vi "DB - Array to Values.vi"(11 "Array (0xFFFE autodetect)":string[](array[string])) -> (3 "<Values>":string)   [LabVIEW 2020]
panel:
  # "abc\ndef\nghi\n(BOM)de"
  # "="
  # "'abc' ,'def' ,'ghi',CONVERT(varbinary(max),'0xFFFE6465',1)"
  # "BOM attached"
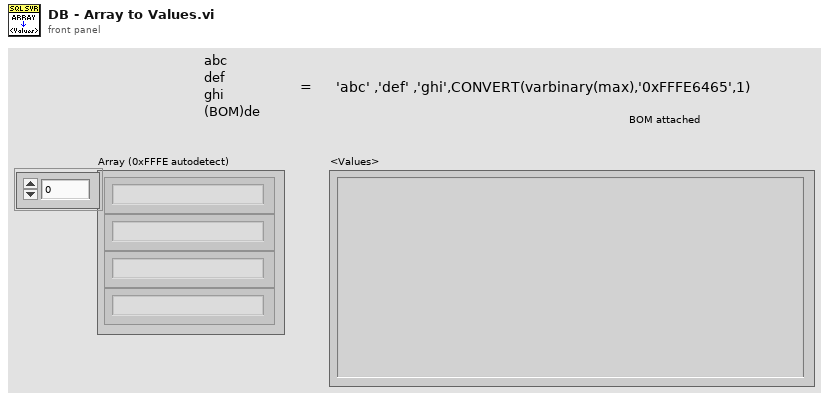
[diagram p1: front panel]
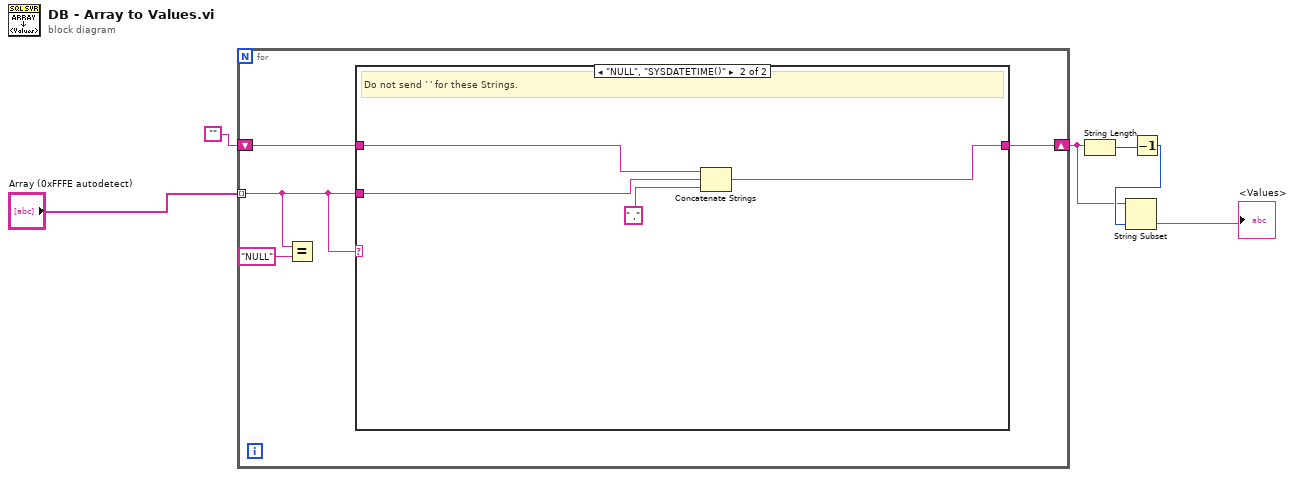
[diagram p0: block diagram]
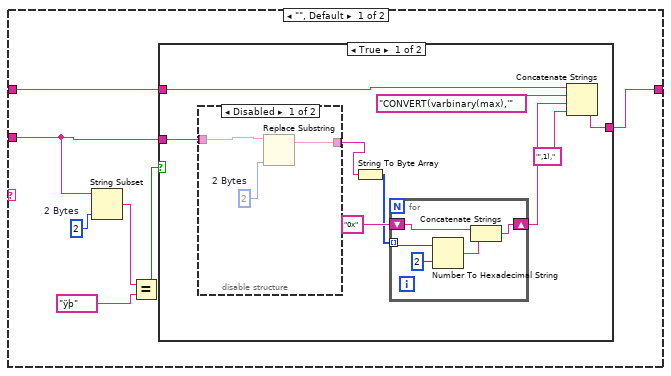
[diagram p2: hidden frame]
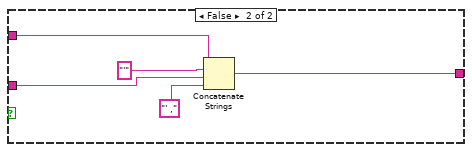
[diagram p4: hidden frame]
diagram:
  n1 = for {
    shift-right: [w9] -> w2
    shift-left: "" -> [w10]
    tunnel: "Array (0xFFFE autodetect)" -> [w7] mode=indexing
    n2 = Equal?(x=w7, y="NULL") -> ()  [unwired: 1 out]
    n3 = case shown="\"NULL\", \"SYSDATETIME()\"" w7 {
      tunnel: w10 -> [w17 w44]
      tunnel: [w16 w42] -> w9
      tunnel: w7 -> [w15 w41]
      frame "", Default {
        w14 = 2  # 2 Bytes
        n4 = String Subset(string=w15, length (rest)=w14) -> (substring=w13:string)  [unwired: 1 in]
        n5 = Equal?(x=w13, y="ÿþ" ("search string")) -> (x = y?=w11:bool)
        n6 = case shown="True" w11 {
          tunnel: w17 -> [w21 w40]
          tunnel: [w18 w38] -> w16
          tunnel: w15 -> [w26 w36]
          frame True {
            n7 = disable-structure shown="Disabled" {
              disable-tunnel: w26 -> [w29 w30]
              disable-tunnel: [w27 w30] -> w22
              frame Disabled {
                w28 = 2  # 2 Bytes
                n8 = Replace Substring(2:w28, 5:w29) -> (1:w27:string)  [unwired: 2 in, 1 out]
              }
              frame Enabled {
              }
            }
            n9 = String To Byte Array(string=w22) -> (unsigned byte array=w23:u8[])
            n10 = for {
              tunnel: w23 -> [w35] mode=indexing
              shift-right: [w33] -> w20
              shift-left: "0x" -> [w32]
              n11 = Number To Hexadecimal String(1:i16 2 ("width (-)"), 2:w35) -> (0:w34:string)
              n12 = Concatenate Strings(w32, w34) -> (w33:string)
            }
            n13 = Concatenate Strings(w21, "CONVERT(varbinary(max),'" ("string"), w20, "',1)," ("string")) -> (w18:string)
          }
          frame False {
            n14 = Concatenate Strings(w40, "'", w36, "' ,") -> (w38:string)
          }
        }
      }
      frame "NULL", "SYSDATETIME()" {
        # "Do not send ' ' for these Strings."
        n15 = Concatenate Strings(w44, w41, " ,") -> (w42:string)
      }
    }
  }
  n16 = String Length(string=w2) -> (length=w3:i32)
  n17 = Decrement(x=w3) -> (x-1=w4:i32)
  n18 = String Subset(string=w2, length (rest)=w4) -> (substring=→"<Values>":string)  [unwired: 1 in]
